vi "Read Mode Command (Single).vi"(8 "error in":errorcluster, 9 "Channel Index":i32=1, 11 "Control Mode in":refnum<class "Control Mode.lvclass">) -> (0 "error out":errorcluster, 1 "Changed or First Call?":bool, 2 "Mode":T1=1 items=["Constant Current"=1, "Constant Voltage"=2, "Battery Emulator"=100, "Fuel Cell Emulator"=101], 3 "Control Mode out":refnum<class "Control Mode.lvclass">)   [LabVIEW 2023, in "Control Mode.lvclass"]
uses:
  Control Mode.lvclass
  Mode.ctl
  Control Mode.lvclass/Control Mode.ctl
  <vilib>/ADAS Replay HIL/Channels/Tag Wrapper/Polymorphic/Read Channel (U32).vi
  <vilib>/ADAS Replay HIL/Channels/Tag Wrapper/Polymorphic/Read Channel (U32).vi/b2f764de-0c1e-4784-a155-687fc995a684.vi
  <vilib>/ADAS Replay HIL/Channels/Tag Wrapper/Polymorphic/Read Channel (U32).vi/b2f764de-0c1e-4784-a155-687fc995a684.vi/c28b0ead-42ad-4072-80a2-aca7f2bd7ce3.vi
  <vilib>/ADAS Replay HIL/Channels/Tag Wrapper/Polymorphic/Read Channel (U32).vi/b2f764de-0c1e-4784-a155-687fc995a684.vi/219d0231-d98b-4193-b5cc-84f90e3c9091.vi
  <vilib>/ADAS Replay HIL/Channels/Tag Wrapper/Tag Wrapper.lvlib
  cdc4fb7e-80ce-4fe1-b86e-a868692c375b.vi
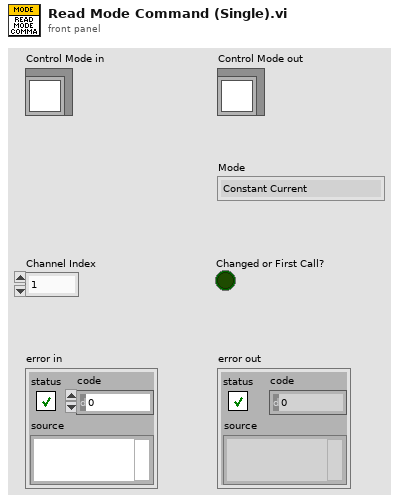
[diagram p1: front panel]
types:
  T1 = typedef "Control Mode.lvclass/Mode.ctl" = u32
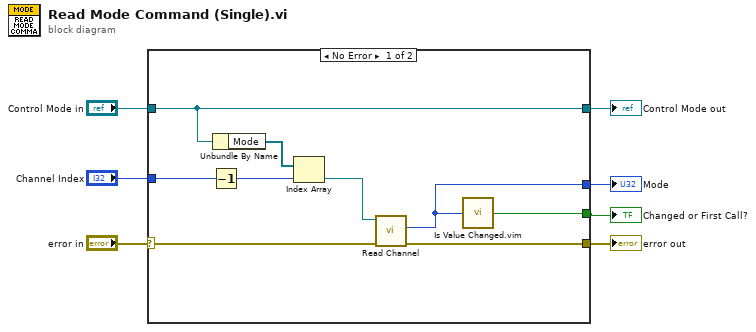
[diagram p0: block diagram]
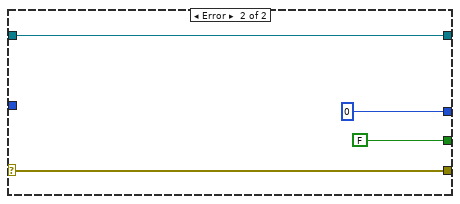
[diagram p2: hidden frame]
diagram:
  n1 = case shown="No Error" "error in" {
    selector: "error in" -> [w15 w20]
    tunnel: [w14 w20] -> w6
    tunnel: [w16 w19] -> w4
    tunnel: "Control Mode in" -> [w16 w19]
    tunnel: [w9 u32 0] -> w3
    tunnel: "Channel Index" -> [w11 _]
    tunnel: [w8 FALSE ("changed or first call?")] -> w1
    frame No Error {
      n2 = Decrement(x=w11) -> (x-1=w10:i32)
      n3 = Unbundle By Name(w16) -> ("Mode"=w13:refnum<k21>[])
      n4 = Index Array(array=w13, index=w10) -> (element=w12:refnum<k21>)
      n5 = call-poly <vilib>:"Read Channel.vi"("error in"=w15, "ADAS HIL Channel in"=w12) -> ("error out"=w14:errorcluster, "Value out"=w9:u32)  [unwired: 6 in, 2 out]
      n6 = call "Is Value Changed.vim"("value"=w9) -> ("changed or first call?"=w8:bool)
    }
    frame Error {
    }
  }
  "error out" <- w6
  "Control Mode out" <- w4
  "Mode" <- w3
  "Changed or First Call?" <- w1
